vi "Complex Determinant.vi"(2 "matrix type":T1(ring), 3 "Input Matrix":T2) -> (0 "error":i32, 1 "determinant":cdb format="%.2e")   [LabVIEW 2020, in "NI_AALBase.lvlib"]
doc: "Computes the <B>determinant</B> of <B>Input Matrix</B>. Wire data to the <B>Input Matrix</B> input to determine the polymorphic instance to use or manually select the instance."
uses:
  <vilib>/Analysis/NI_AALBase.lvlib
  <vilib>/Analysis/Matrix/Datatypes/ComplexMatrix.ctl
  <resource>/lvanlys.dll
  <vilib>/Analysis/Matrix/NI_Matrix.lvlib
panel:
  # "Complex Determinant"
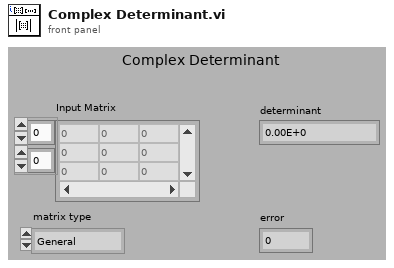
[diagram p1: front panel]
types:
  T1 = enum32{"General", "Positive Definite", "Lower Triangular", "Upper Triangular"}
  T2 = typedef "NI_Matrix.lvlib/ComplexMatrix.ctl" = cdb[][]
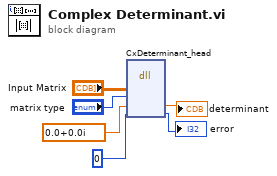
[diagram p0: block diagram]
diagram:
  n1 = dll-call lib="e:/builds/penguin/labview/branches/2020/dev/dist/resource/lvanlys.*" fn="CxDeterminant_head"("Input Matrix"="Input Matrix", "matrix type"="matrix type", cdb 0.0+0.0i, 0) -> (→"determinant":cdb, →"error":i32)  [unwired: 6 in, 2 out]
